vi "Destroy.vi"(8 "error in (no error)":errorcluster, 11 "WorkTable Class.lvclass":refnum<class "WorkTable Class.lvclass">) -> (0 "error out":errorcluster)   [LabVIEW 2011, in "WorkTable Class.lvclass"]
uses:
  WorkTable Class.lvclass
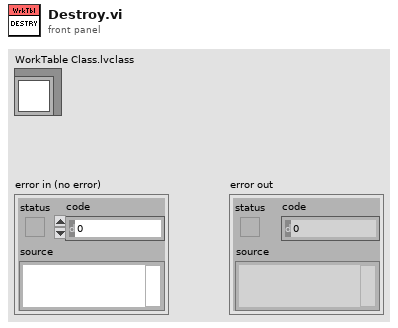
[diagram p1: front panel]
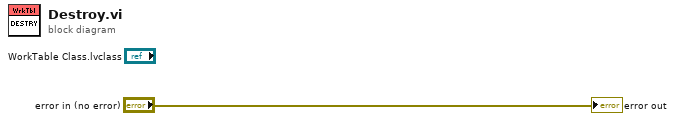
[diagram p0: block diagram]
diagram:
  "error out" <- "error in (no error)"
